vi "Soft_Robot_Model_State Estimator.vi"() -> ()   [LabVIEW 2015]
uses:
  <vilib>/rvi/interface/nirviReadWriteControl/nirviReadWriteControl.xnode
  <vilib>/Utility/error.llb/Error Cluster From Error Code.vi
  <vilib>/rvi/errors/niLvFpgaAdjustHostInterfaceError.vi
  <vilib>/rvi/interface/nirviCloseFPGA/nirviCloseFPGA.xnode
  <vilib>/addons/Control Design/_Model Construction/NI_LinSys_Model Creation.lvlib
  <vilib>/Simulation/Implementation/XNodeFramework/SimXNode/SimX.xnode
  <vilib>/addons/Control Design/_Stochastic Systems/NI_CD_Stochastic Systems.lvlib
  <vilib>/rvi/interface/nirviOpenFPGA/nirviOpenFPGA.xnode
  <vilib>/addons/Control Design/_Model Construction/Model Creation.llb/Model Creation SubVI/cd_Create State Space Model.vi
  <vilib>/Platform/TimedLoop/XDataNode/XDataNode.xnode
  <vilib>/Platform/TimedLoop/XDataNode/nitl_modes.ctl
  <vilib>/Platform/TimedLoop/XDataNode/XDNodeRunTimeDep.lvlib
  <vilib>/Platform/TimedLoop/XDataNode/wakeup.ctl
  <vilib>/Platform/TimedLoop/XDataNode/timing_clust.ctl
  FPGA Bitfiles/ACC20115_FPGATarget_CurrentControlle_Dt5vFgOzYtY.lvbitx
  Current Controller.vi
  <vilib>/FPGAPlugInAG/myRIO-1900/niLvFpga_Open_myRIO-1900.vi
  <vilib>/rvi/interface/common/dynamic/niFpgaDynamicAddResources.vi
  NiFpgaLv.dll
  <vilib>/rvi/interface/Simulation/niFpgaSimulationCallBeginRW.vi
  <vilib>/FPGAPlugInAG/Dynamic/niLvFpga_Close_Dynamic.vi
  <vilib>/addons/Control Design/_State Feedback Control/NI_CD_State Feedback Control.lvlib
  <vilib>/addons/Control Design/_State Feedback Control/State Feedback Control.llb/CD State Compensator.vi
  <vilib>/Simulation/Estimation/Implementation/NILVSim Discrete Kalman Filter.llb/SIM Disc KF Pred and Corr with Pred Gain with Checking Direct LV.vi
  <vilib>/addons/Control Design/_Stochastic Systems/Stochastic Systems.llb/Stochastic Systems SubVIs/cd_Stochastic State-Space Model.ctl
  <vilib>/addons/Control Design/_Stochastic Systems/Stochastic Systems.llb/Stochastic Systems SubVIs/cd_Second-Order Statistics Noise Model.ctl
  <vilib>/addons/Control Design/_State Feedback Control/State Feedback Control.llb/State Feedback Control SubVis/cd_State Estimator Single Output.vi
  <vilib>/addons/Control Design/_Model Construction/Model Typedefs.llb/CD General Elements.ctl
  <vilib>/addons/Control Design/_Model Construction/NI_LinSys_Model Typedefs.lvlib
  <vilib>/addons/Control Design/_Model Construction/Model Typedefs.llb/CD State Space Model (MIMO).ctl
panel:
  in  "SP1: 2":dbl(slide)=40.87020302841148 min=0.0 max=0.0 scale=0.0..720.0
  in  "Tab Control":enum32{"Outputs", "Inputs"}(tab)
  out "Fusion Data":dbl(graph)
  out "KF estimate":dbl[](graph)
  in  "Stop":bool
  out "DAC Inlet Valve 2":i32(graph)
  in  "Current (mA)":i32
  out "Status?":bool
  out "State-Space Model":T1 {"Transport Delay" format="%.2f"; "D" format="%#.2g"; "C" format="%#.2g"; "B" format="%#.2g"; "A" format="%#.2g"; "properties"."Sampling Time" format="%#.6p"; "properties"."Output Delays" format="%.4f"; "properties"."Input Delays" format="%.4f"}
  out "Kalman Filter Gain M(k)":dbl[][](array[numeric])
  in  "A":dbl[][](array[numeric]) format="%#.5g"
  in  "B":dbl[][](array[numeric]) format="%#.5g"
  in  "C":dbl[][](array[numeric]) format="%#.5g"
  in  "G":dbl[][](array[numeric]) format="%#.2g"
  out "error out":errorcluster
  in  "Desired CL Poles":cdb[](array[numeric]) format="%.3f"
  out "Actual CL Poles":cdb[](array[numeric]) format="%.3f"
  out "LQR Error":errorcluster
  out "KF Error":errorcluster
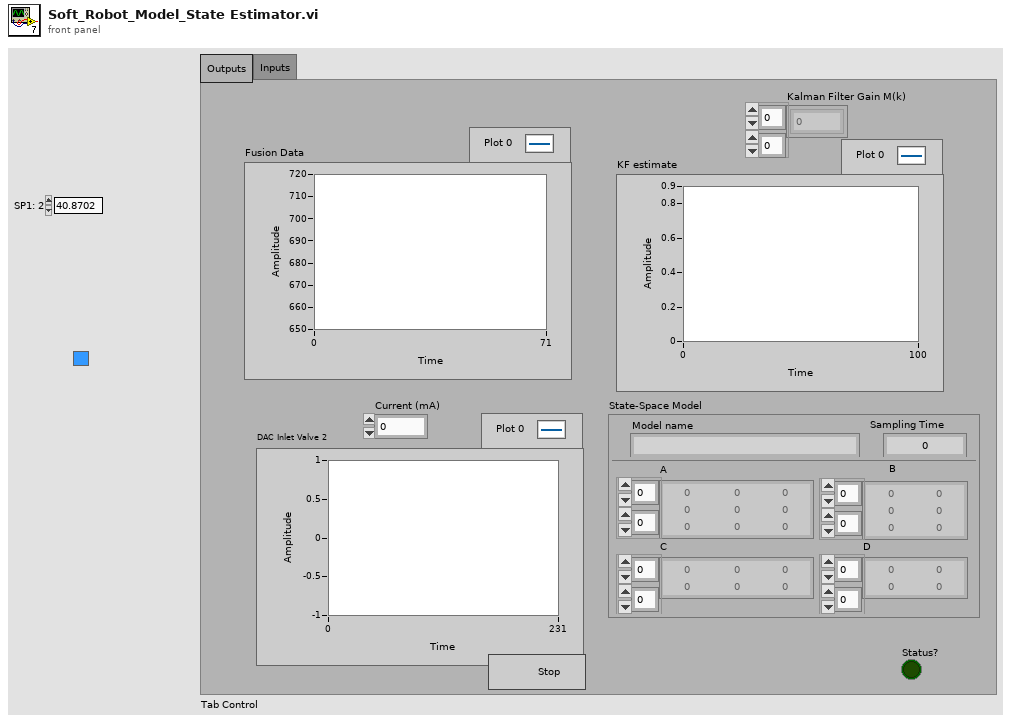
[diagram p1: front panel]
types:
  T1 = typedef "NI_LinSys_Model Typedefs.lvlib/CD State Space Model (MIMO).ctl" = cluster{"properties":T2, "A":dbl[][], "B":dbl[][], "C":dbl[][], "D":dbl[][], "StateNames":string[], "Transport Delay":dbl[][]}
  T2 = typedef "NI_LinSys_Model Typedefs.lvlib/CD General Elements.ctl" = cluster{"Model name":string, "Input names":string[], "Output names":string[], "Input Delays":dbl[], "Output Delays":dbl[], "Sampling Time":dbl, "Notes":string}
  T3 = typedef "XDNodeRunTimeDep.lvlib/timing_clust.ctl" = cluster{"Expected End [f-1]":u64, "Actual End [f-1]":u64, "Finished Late? [f-1]":bool, "Expected End [i-1]":u64, "Actual End [i-1]":u64, "Finished Late? [i-1]":bool, "Expected Start [i]":u64, "Actual Start [i]":u64, "Expected Start [f]":u64, "Actual Start [f]":u64, "Source Name":string, "Structure Name":string, "Period":i64, "Deadline":i64, "Offset":i64, "Start":i64, "Priority":i32, "Timeout":i32, "Mode":T4, "Wakeup Reason":T5, "Error":errorcluster, "Source Type":string, "Secondary Source Type":string, "Global End Time":u64, "Global Start Time":u64, "Frame Duration":u64, "Iteration Duration":u64, "Assigned CPU":i32, "I/O Scan Engine Mode":u32}
  T4 = typedef "XDNodeRunTimeDep.lvlib/nitl_modes.ctl" = enum32{"No Change", "Process missed periods, maintain original phase", "Discard missed periods, maintain original phase", "Process missed periods, ignore original phase", "Discard missed periods, ignore original phase"}
  T5 = typedef "XDNodeRunTimeDep.lvlib/wakeup.ctl" = enum32{"Normal", "Aborted", "Asynchronous wakeup", "Timing source error", "Timed loop error", "Timeout"}
  T6 = enum16{"System Included", "System Included with Noise", "Standalone"}
  T7 = typedef "NI_CD_Stochastic Systems.lvlib/cd_Second-Order Statistics Noise Model.ctl" = cluster{"Q":dbl[][], "E{w}":dbl[], "E{v}":dbl[], "R":dbl[][], "N":dbl[][]}
  T8 = typedef "NI_CD_Stochastic Systems.lvlib/cd_Stochastic State-Space Model.ctl" = cluster{"Sampling Time (s)":dbl, "G":dbl[][], "B":dbl[][], "A":dbl[][], "C":dbl[][], "D":dbl[][], "H":dbl[][]}
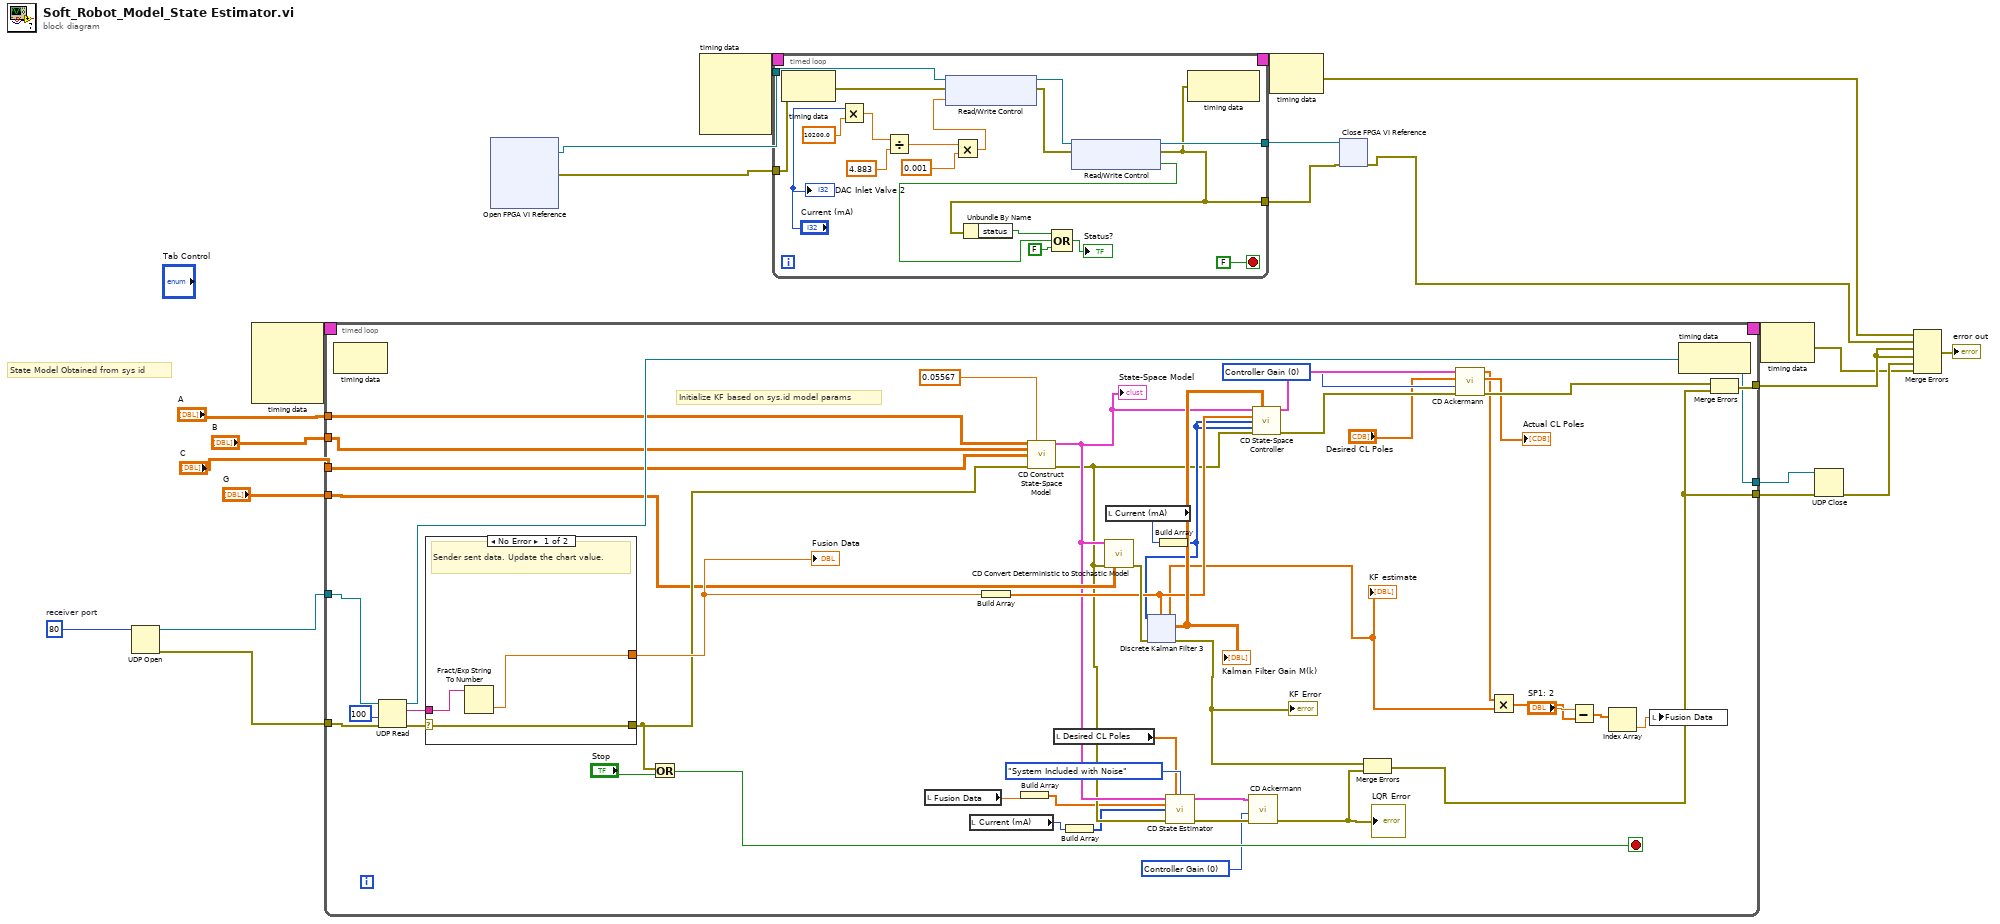
[diagram p0: block diagram]
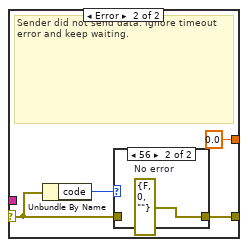
[diagram p2: hidden frame]
diagram:
  w21 = u16 80  # receiver port
  # "State Model Obtained from sys id"
  n1 = UDP Open(11:w21) -> (port=w20:refnum<k16>, 0:w19:errorcluster)  [unwired: 4 in, 1 out]
  n2 = node-c288() -> (w11:T3)  [unwired: 4 in]
  n3 = timed-loop {
    tunnel: [w67] -> w16
    tunnel: w20 -> [w62]
    tunnel: w19 -> [w61]
    tunnel: [w58] -> w18
    tunnel: "A" -> [w57]
    tunnel: "B" -> [w56]
    tunnel: "C" -> [w55]
    timing: w11 -> [_]
    timing-out: [_] -> w10
    tunnel: "G" -> [w52]
    tunnel: [w50] -> w2
    stop <- w59 stop-if-true
    w24 = u16 0 items=["Controller Gain", "Observer Gain (Predictive)", "Observer Gain (Current)"] ("Gain Type")
    w44 = u16 0 items=["Controller Gain", "Observer Gain (Predictive)", "Observer Gain (Current)"] ("Gain Type")
    # "Initialize KF based on sys.id model params"
    n4 = node-c288() -> ()  [unwired: 1 in, 1 out]
    n5 = UDP Read(connection ID=w62, timeout ms (25000)=100, 8:w61) -> (data out=w64:string, error out=w63:errorcluster, 3:w58:refnum<k16>)  [unwired: 3 out]
    n6 = case shown="No Error" w63 {
      selector: w63 -> [w74 w78]
      tunnel: w64 -> [w75 _]
      tunnel: [w74 w77] -> w54
      tunnel: [w73 0.0] -> w60
      frame No Error {
        # "Sender sent data. Update the chart value."
        n7 = Fract/Exp String To Number(string=w75) -> (number=w73:dbl)  [unwired: 3 in, 1 out]
      }
      frame Error {
        # "Sender did not send data. Ignore timeout error and keep waiting."
        n8 = Unbundle By Name(w78) -> ("code"=w79:i32)
        n9 = case shown="56" w79 {
          tunnel: w78 -> [w80 _]
          tunnel: [w80 w81] -> w77
          frame Default {
          }
          frame 56 {
            w81 = errorcluster {"status"=FALSE, "code"=0, "source"=""}  # No error
          }
        }
      }
    }
    "Fusion Data" <- w60
    n10 = Or(x=w54, y="Stop") -> (x .or. y?=w59:bool)
    n11 = local read "Fusion Data"() -> (w32:dbl)
    n12 = local read "Current (mA)"() -> (w30:i32)
    n13 = Build Array ("Build Array 6")(w60) -> (w48:dbl[])
    n14 = Build Array(w32) -> (w31:dbl[])
    n15 = call-poly <vilib>:"CD Construct State-Space Model.vi"("A"=w57, "Sampling Time (s)"=0.05567, "B"=w56, "C"=w55, "error in (no error)"=w54) -> ("State-Space Model"=w35:T1, "error out"=w34:errorcluster)  [unwired: 9 in]
    "State-Space Model" <- w35
    n16 = local read "Desired CL Poles"() -> (w26:cdb[])
    n17 = Build Array(w30) -> (w29:i32[])
    n18 = call <vilib>:"CD Convert Deterministic to Stochastic Model.vi"("Deterministic State-Space Model"=w35, "error in (no error)"=w34, "G"=w52) -> ("error out"=w53:errorcluster)  [unwired: 11 in, 1 out]
    n19 = local read "Current (mA)"() -> (w69:i32)
    n20 = Build Array ("Build Array 5")(w69) -> (w47:i32[])
    n21 = xnode ("Discrete Kalman Filter 3")("input u(k)"=w47, "Output y(k)"=w48, "error in (no error)"=w53) -> ("Estimated Output yhat(k)"=w39:dbl[], "Kalman Filter Gain M(k)"=w49:dbl[][], "error out"=w68:errorcluster)  [unwired: 5 out]
    "KF estimate" <- w39
    "Kalman Filter Gain M(k)" <- w49
    "KF Error" <- w68
    n22 = call-poly <vilib>:"CD State Estimator.vi"("State-Space Model"=w35, "Estimator Gain (L)"=w26, "Configuration"=T6."System Included with Noise", "Measured Outputs"=w31, "Known Inputs"=w29, "error in (no error)"=w34) -> ("Estimator Model"=w27:T1, "error out"=w28:errorcluster)  [unwired: 8 in]
    n23 = call <vilib>:"CD Ackermann.vi"("error in (no error)"=w28, "Gain Type"=w24, "State-Space Model"=w27) -> ("error out"=w25:errorcluster)  [unwired: 6 in, 2 out]
    "LQR Error" <- w25
    n24 = call-poly <vilib>:"CD State-Space Controller.vi"("State-Space Model"=w35, "Estimator Gain (L)"=w49, "Measured Outputs"=w48, "Known Inputs"=w47, "Manipulated Inputs"=w47, "error in (no error)"=w34) -> ("Controller Model"=w46:T1, "error out"=w45:errorcluster)  [unwired: 8 in]
    n25 = Merge Errors(w68, w25) -> (w50:errorcluster)
    n26 = call <vilib>:"CD Ackermann.vi"("error in (no error)"=w45, "Gain Type"=w44, "Poles"="Desired CL Poles", "State-Space Model"=w46) -> ("error out"=w43:errorcluster, "Actual Poles"=→"Actual CL Poles":cdb[], "Gain"=w40:dbl[])  [unwired: 5 in]
    n27 = Multiply(x=w40, y=w39) -> (x*y=w38:dbl[])
    n28 = Subtract(x="SP1: 2", y=w38) -> (x-y=w37:dbl[])
    n29 = Index Array(array=w37) -> (element=w36:dbl)  [unwired: 1 in]
    n30 = local write "Fusion Data"(w36) -> ()
    n31 = node-c288() -> ()  [unwired: 1 in, 1 out]
    n32 = Merge Errors(w43, w50) -> (w67:errorcluster)
  }
  n33 = xnode "Open FPGA VI Reference"() -> ("FPGA VI Reference Out"=w8:refnum<k20>, "error out"=w7:errorcluster)  [unwired: 2 in]
  n34 = node-c288() -> (w6:T3)  [unwired: 4 in]
  n35 = timed-loop {
    tunnel: w8 -> [w113]
    tunnel: w7 -> [w98]
    tunnel: [w97] -> w22
    tunnel: [w106] -> w23
    timing: w6 -> [_]
    timing-out: [_] -> w5
    stop <- FALSE stop-if-true
    n36 = node-c288() -> ()  [unwired: 1 in, 1 out]
    n37 = Multiply(x="Current (mA)", y=10200.0) -> (x*y=w101:dbl)
    n38 = Divide(x=w101, y=4.883) -> (x/y=w104:dbl)
    n39 = Multiply(x=w104, y=0.001) -> (x*y=w100:dbl)
    n40 = xnode "Read/Write Control"("FPGA VI Reference In"=w113, "error in"=w98, "DAC Inlet Valve"=w100) -> ("FPGA VI Reference Out"=w112:refnum<k20>, "error out"=w111:errorcluster)
    n41 = xnode "Read/Write Control"("FPGA VI Reference In"=w112, "error in"=w111) -> ("FPGA VI Reference Out"=w106:refnum<k20>, "error out"=w97:errorcluster, "Inlet Overflow?"=w107:bool)
    n42 = Unbundle By Name(w97) -> ("status"=w109:bool)
    n43 = Compound Arithmetic op=OR(w109, w107, FALSE ("value")) -> (→"Status?":bool)
    n44 = node-c288(w97) -> ()  [unwired: 1 out]
    "DAC Inlet Valve 2" <- "Current (mA)"
  }
  n45 = node-c288(w5) -> (w3:errorcluster)
  n46 = xnode "Close FPGA VI Reference"("FPGA VI Reference In"=w23, "error in"=w22) -> ("error out"=w4:errorcluster)
  n47 = node-c288(w10) -> (w1:errorcluster)
  n48 = UDP Close(connection ID=w18, 8:w2) -> (error out=w17:errorcluster)  [unwired: 1 out]
  n49 = Merge Errors(w3, w4, w16, w16, w17, w1) -> (→"error out":errorcluster)
